vi "APC_WarningColorMap.vi"(1 "Array":u8[](array[numeric])) -> (0 "Round Color Box":u32[](array[colorbox]))   [LabVIEW 2020]
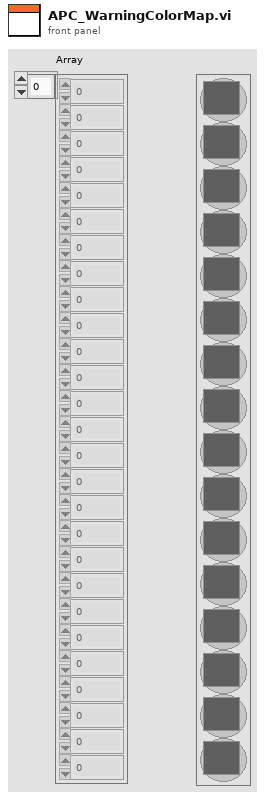
[diagram p1: front panel]
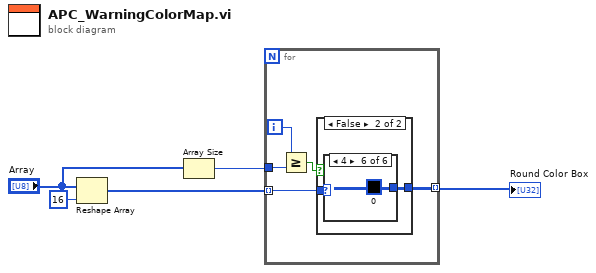
[diagram p0: block diagram]
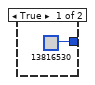
[diagram p2: hidden frame]
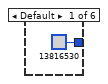
[diagram p3: hidden frame]
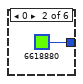
[diagram p4: hidden frame]
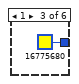
[diagram p5: hidden frame]
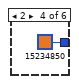
[diagram p6: hidden frame]
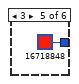
[diagram p7: hidden frame]
diagram:
  n1 = Reshape Array("Array", 16 ("dimension size")) -> (w4:u8[])
  n2 = Array Size(array="Array") -> (size(s)=w2:i32)
  n3 = for {
    tunnel: [w10] -> w1 mode=indexing
    tunnel: w4 -> [w9] mode=indexing
    tunnel: w2 -> [w7]
    i -> [w6]
    n4 = Greater Or Equal?(x=w6, y=w7) -> (x >= y?=w8:bool)
    n5 = case shown="False" w8 {
      tunnel: [u32 13816530 ("Round Color Box") w13] -> w10
      tunnel: w9 -> [_ w12]
      frame True {
      }
      frame False {
        n6 = case shown="4" w12 {
          tunnel: [u32 13816530 ("Round Color Box") u32 6618880 ("Round Color Box") u32 16775680 ("Round Color Box") u32 15234850 ("Round Color Box") u32 16718848 ("Round Color Box") u32 0 ("Round Color Box")] -> w13
          frame Default {
          }
          frame 0 {
          }
          frame 1 {
          }
          frame 2 {
          }
          frame 3 {
          }
          frame 4 {
          }
        }
      }
    }
  }
  "Round Color Box" <- w1
